vi "Teleop.vi"(10 "Match Info":T2={"Autonomous Elapsed Seconds"=0.0, "TeleOp Elapsed Seconds"=0.0, "Disabled Elapsed Seconds"=0.0, "Visited Autonomous"=FALSE, "Visited TeleOp"=FALSE, "Visited Disabled"=FALSE, "Autonomous Settings"={"Autonomous Style"=enum."Independent", "VI Refnum"=refnum}}, 11 "Call Context":T3) -> ()   [LabVIEW 2016]
doc: "This VI is called for each TeleOp packet received from the DS where the robot is not disabled. It is often used to read from the joysticks and update I/O or to update setpoints for timed control loops. It should complete and return within 20 milliseconds or it may miss DS packets."
uses:
  <vilib>/Rock Robotics/WPI/DriverStation/WPI_DriverStationDerivedRobotMode.ctl
  <vilib>/Rock Robotics/WPI/DriverStation/WPI_DriverStationMatch Info.ctl
  <vilib>/Rock Robotics/Network Tables/NT Read Boolean.vi
  <vilib>/Rock Robotics/Network Tables/NT Read Number.vi
  <vilib>/Rock Robotics/WPI/Utilities/WPI_GetSetVariantRefNum.vi
panel:
  in  "Servo":T1
  out "Sample Slider 0":dbl(slide) scale=0.0..5.0
  out "Sample Boolean 1":bool
  out "Sample Boolean 0":bool
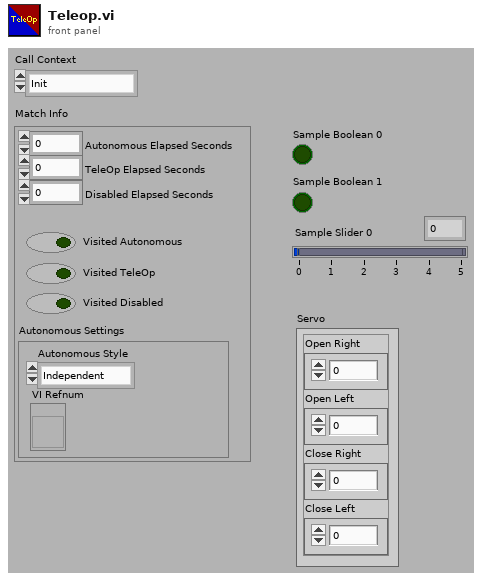
[diagram p1: front panel]
types:
  T1 = cluster{"Open Right":dbl, "Open Left":dbl, "Close Right ":dbl, "Close Left":dbl}
  T2 = typedef "WPI_DriverStationMatch Info.ctl" = cluster{"Autonomous Elapsed Seconds":dbl, "TeleOp Elapsed Seconds":dbl, "Disabled Elapsed Seconds":dbl, "Visited Autonomous":bool, "Visited TeleOp":bool, "Visited Disabled":bool, "Autonomous Settings":cluster{"Autonomous Style":enum16{"Iterative", "Independent"}, "VI Refnum":refnum<vi>}}
  T3 = typedef "WPI_DriverStationDerivedRobotMode.ctl" = enum16{"Init", "Execute", "Stop"}
  T4 = cluster{"Joystick Right":dbl, "Joystick Left":dbl, "Keep Pose":bool, "Keep Angle":bool, "Slow Drive":bool, "Drive To Target":bool}
  T5 = typedef "WPI_JoystickDevRef.ctl" = cluster{"Device":T6}
  T6 = typedef "WPI_JoystickDeviceEnum.ctl" = enum16{"USB 0", "USB 1", "USB 2", "USB 3", "USB 4", "USB 5"}
  T7 = cluster{"Axes[0]":dbl, "Axes[1]":dbl, "Axes[2]":dbl, "Axes[3]":dbl, "Axes[4]":dbl, "Axes[5]":dbl, "Axes[6]":dbl, "Axes[7]":dbl, "Axes[8]":dbl}
  T8 = cluster{"Buttons[0]":bool, "Buttons[1]":bool, "Buttons[2]":bool, "Buttons[3]":bool, "Buttons[4]":bool, "Buttons[5]":bool, "Buttons[6]":bool, "Buttons[7]":bool, "Buttons[8]":bool}
  T9 = cluster{"Right Button":bool, "Left Button ":bool, "Y":bool, "B":bool, "A":bool, "X":bool, "Left Stick X":dbl, "Left Stick Y":dbl, "Right Stick X ":dbl, "Right Stick Y ":dbl, "Center Left":bool, "Center Right":bool, "Right Stick Touch":bool, "Left Stick Touch ":bool, "Arrows":i16, "Left Throttle":dbl, "Right Throttle":dbl}
  T10 = typedef "WPI_MotorControlDeviceRef.ctl" = cluster{"DeviceStatus":errorcluster, "Type":T11, "PWM":cluster{"PWM Channel":T12, "DeadBand":T13}, "CAN":cluster{"Device Number":u8, "SetOutput VI Ref":variant, "GetOutput VI Ref":variant, "Enable VI Ref":variant, "Disable VI Ref":variant, "Data":variant}, "Invert":bool}
  T11 = typedef "WPI_MotorControlType.ctl" = enum16{"PWM", "CAN"}
  T12 = typedef "FPGA_DIOPWMChannel.ctl" = enum8{"PWM 0", "PWM 1", "PWM 2", "PWM 3", "PWM 4", "PWM 5", "PWM 6", "PWM 7", "PWM 8", "PWM 9", "PWM MXP 0", "PWM MXP 1", "PWM MXP 2", "PWM MXP 3", "PWM MXP 4", "PWM MXP 5", "PWM MXP 6", "PWM MXP 7", "PWM MXP 8", "PWM MXP 9", "Invalid"}
  T13 = typedef "WPI_PWMDeadband.ctl" = cluster{"Name":string, "maxPositivePwm":i32, "minPositivePwm":i32, "centerPwm":i32, "maxNegativePwm":i32, "minNegativePwm":i32, "angularRange":u16}
  T14 = typedef "WPI_ServoDeviceRef.ctl" = cluster{"DeviceStatus":errorcluster, "PWM Channel":T12, "DeadBand":T13}
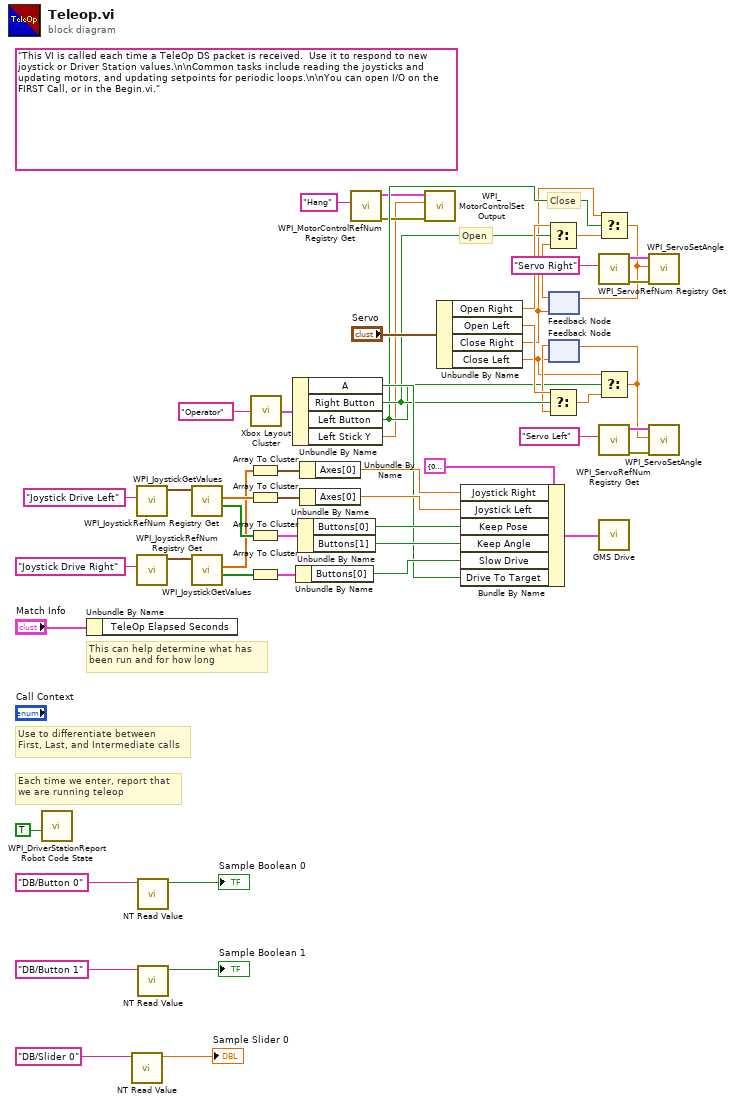
[diagram p0: block diagram]
diagram:
  (unwired) "This VI is called each time a TeleOp DS packet is received.  Use it to respond to new joystick or Driver Station values.\n\nCommon tasks include reading the joysticks and updating motors, and updating setpoints for periodic loops.\n\nYou can open I/O on the FIRST Call, or in the Begin.vi."
  # "Close"
  # "Open"
  # "Each time we enter, report that\nwe are running teleop"
  # "Use to differentiate between\nFirst, Last, and Intermediate calls"
  # "This can help determine what has\nbeen run and for how long"
  n1 = call <vilib>:"WPI_DriverStationReport Robot Code State.vi"("TeleOp"=TRUE ("Autonomous")) -> ()  [unwired: 10 in, 1 out]
  n2 = Unbundle By Name("Match Info") -> ()  [unwired: 1 out]
  n3 = call-poly <vilib>:"NT Read Value.vi"("Name"="DB/Slider 0" ("refnum name")) -> ("Numeric"=→"Sample Slider 0":dbl)  [unwired: 9 in, 1 out]
  n4 = call <vilib>:"WPI_JoystickRefNum Registry Get.vi"("refnum name"="Joystick Drive Left") -> ("JoystickDevRef"=w44:T5)  [unwired: 9 in, 1 out]
  n5 = call <vilib>:"WPI_JoystickRefNum Registry Get.vi"("refnum name"="Joystick Drive Right") -> ("JoystickDevRef"=w36:T5)  [unwired: 9 in, 1 out]
  n6 = call-poly <vilib>:"NT Read Value.vi"("Name"="DB/Button 0" ("refnum name")) -> ("Boolean"=→"Sample Boolean 0":bool)  [unwired: 9 in, 1 out]
  n7 = call-poly <vilib>:"NT Read Value.vi"("Name"="DB/Button 1" ("refnum name")) -> ("Boolean"=→"Sample Boolean 1":bool)  [unwired: 9 in, 1 out]
  n8 = call <vilib>:"WPI_JoystickGetValues.vi"("JoystickDevRef"=w44) -> ("Buttons"=w41:bool[], "Axes"=w42:dbl[])  [unwired: 6 in, 3 out]
  n9 = call <vilib>:"WPI_JoystickGetValues.vi"("JoystickDevRef"=w36) -> ("Buttons"=w31:bool[], "Axes"=w34:dbl[])  [unwired: 6 in, 3 out]
  n10 = Array To Cluster(array=w34) -> (cluster=w33:T7)
  n11 = Array To Cluster(array=w42) -> (cluster=w43:T7)
  n12 = Array To Cluster(array=w41) -> (cluster=w40:T8)
  n13 = Array To Cluster(array=w31) -> (cluster=w30:T8)
  n14 = call "Xbox Layout Cluster.vi"("Joystick Name"="Operator") -> ("Joystick Out"=w25:T9)
  n15 = Unbundle By Name(w25) -> ("A"=w24:bool, "Right Button"=w12:bool, "Left Button"=w9:bool, "Left Stick Y"=w1:dbl)
  n16 = Unbundle By Name(w30) -> ("Buttons[0]"=w27:bool)
  n17 = Unbundle By Name(w40) -> ("Buttons[0]"=w29:bool, "Buttons[1]"=w28:bool)
  n18 = Unbundle By Name(w33) -> ("Axes[0]"=w32:dbl)
  n19 = Unbundle By Name(w43) -> ("Axes[0]"=w37:dbl)
  n20 = call <vilib>:"WPI_MotorControlRefNum Registry Get.vi"("refnum name"="Hang") -> ("error out"=w4:errorcluster, "MotorControlDevRef"=w3:T10)  [unwired: 9 in]
  n21 = call <vilib>:"WPI_MotorControlSetOutput.vi"("error in (no error)"=w4, "Output"=w1, "MotorControlDevRef"=w3) -> ()  [unwired: 6 in, 3 out]
  n22 = Unbundle By Name("Servo") -> ("Open Right"=w14:dbl, "Open Left"=w11:dbl, "Close Right"=w7:dbl, "Close Left"=w8:dbl)
  n23 = Bundle By Name(cluster=T4 {"Joystick Right"=0.0, "Joystick Left"=0.0, "Keep Pose"=FALSE, "Keep Angle"=FALSE, "Slow Drive"=FALSE, "Drive To Target"=FALSE} ("Joystic Data"), "Joystick Right"=w32, "Joystick Left"=w37, "Keep Pose"=w29, "Keep Angle"=w28, "Slow Drive"=w27, "Drive To Target"=w24) -> (w38:T4)
  n24 = feedback #1(w7) -> (w15:dbl)
  n25 = Select(t=w14, s=w12, f=w15) -> (s? t:f=w16:dbl)
  n26 = feedback #2(w8) -> (w10:dbl)
  n27 = Select(t=w11, s=w12, f=w10) -> (s? t:f=w13:dbl)
  n28 = Select(t=w7, s=w9, f=w16) -> (s? t:f=w6:dbl)
  n29 = feedback-in #1(w6) -> ()
  n30 = call <vilib>:"WPI_ServoRefNum Registry Get.vi"("refnum name"="Servo Right") -> ("error out"=w20:errorcluster, "ServoDeviceRef"=w21:T14)  [unwired: 9 in]
  n31 = Select(t=w8, s=w9, f=w13) -> (s? t:f=w5:dbl)
  n32 = feedback-in #2(w5) -> ()
  n33 = call <vilib>:"WPI_ServoRefNum Registry Get.vi"("refnum name"="Servo Left") -> ("error out"=w23:errorcluster, "ServoDeviceRef"=w22:T14)  [unwired: 9 in]
  n34 = call "GMS Drive.vi"("Joystic Data"=w38) -> ()  [unwired: 1 in]
  n35 = call <vilib>:"WPI_ServoSetAngle.vi"("error in (no error)"=w20, "Angle"=w6, "ServoDeviceRef"=w21) -> ()  [unwired: 7 in, 2 out]
  n36 = call <vilib>:"WPI_ServoSetAngle.vi"("error in (no error)"=w23, "Angle"=w5, "ServoDeviceRef"=w22) -> ()  [unwired: 7 in, 2 out]
